vi "AA CH_LM App Main.vi"() -> ()   [LabVIEW 2012, in "CH_LM App.lvlib"]
doc: "This is the Main.vi of the LabMax PC Application."
uses:
  CH_LM App.lvlib
  CH_LM.lvlib
  CH_LM App FGV Functions.ctl
  _CH_LM/CH_LM FGV Functions.ctl
  CH_LM Globals Debug-Status.vi
panel:
  out "error":errorcluster
  in  "stop":bool
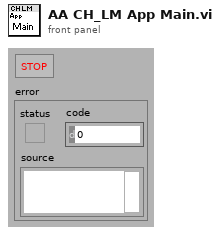
[diagram p1: front panel]
types:
  T1 = typedef "CH_LM.lvlib/CH_LM FGV Functions.ctl" = enum16{"create", "get", "set", "remove", "clear", "getBySerial"}
  T2 = typedef "CH_LM App.lvlib/CH_LM App FGV Functions.ctl" = enum16{"create", "get", "set", "remove", "clear", "getBySerial"}
  T3 = enum32{"Invalid", "Standard", "Closed", "Hidden", "Minimized", "Maximized"}
  T4 = enum32{"invalid app kind", "Development System", "Run Time System", "Student Edition", "Embedded LabVIEW", "Evaluation", "Custom"}
  T5 = typedef "LVRectTypeDef.ctl" = cluster{"Left":i16, "Top":i16, "Right":i16, "Bottom":i16}
  T6 = typedef "CH_LM.lvlib/CH_LM Communication Mode.ctl" = enum16{"None", "USB", "GPIB", "RS232"}
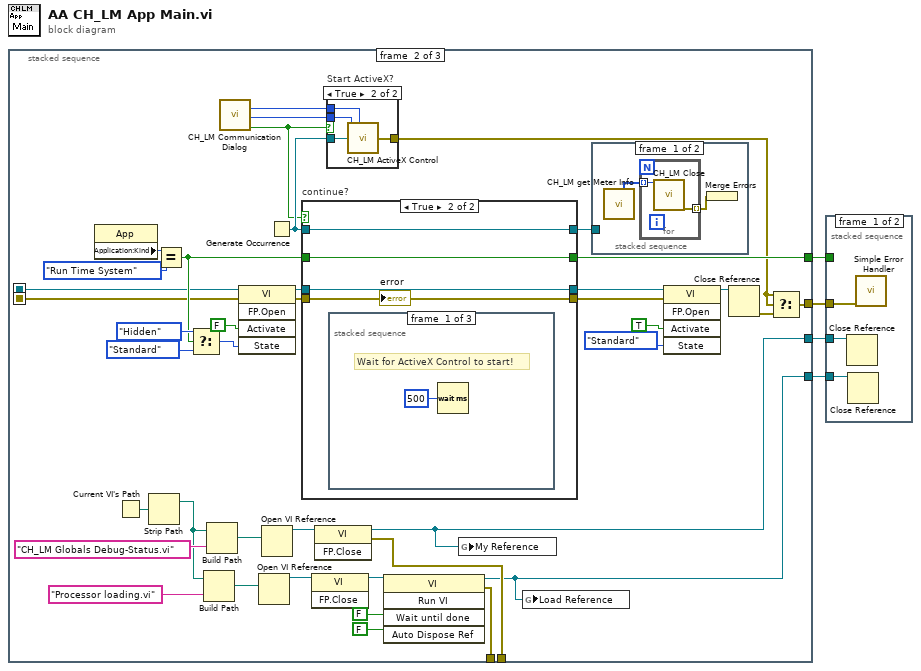
[diagram p0: block diagram]
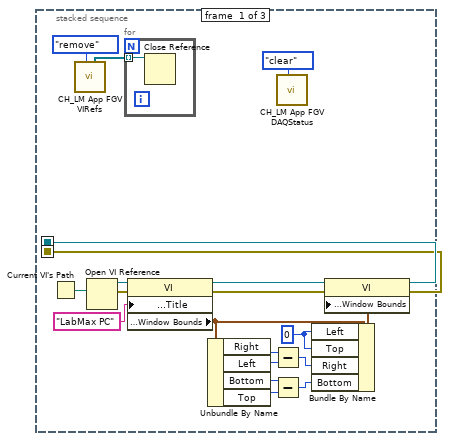
[diagram p2: hidden frame]
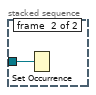
[diagram p3: hidden frame]
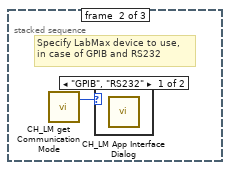
[diagram p6: hidden frame]
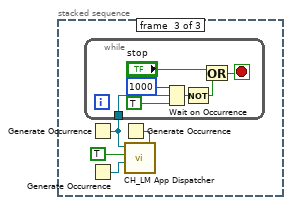
[diagram p8: hidden frame]
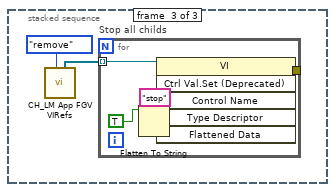
[diagram p9: hidden frame]
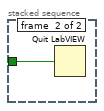
[diagram p10: hidden frame]
diagram:
  n1 = stacked-sequence {
    seq-local: [w15 _ _] -> [_ w43 _]
    seq-local: [w14 _ _] -> [_ w42 _]
    tunnel: [_ w62 _] -> w4
    tunnel: [_ w51 _] -> w3
    tunnel: [_ w36 _] -> w2
    tunnel: [_ w29 _] -> _
    tunnel: [_ w27 _] -> w1
    tunnel: [_ w28 _] -> _
    frame #0 {
      w6 = i16 0 ("left")
      n2 = Current VI's Path() -> (path=w18:path)
      n3 = call "CH_LM App FGV VIRefs.vi"("Function"=CH_LM_App_FGV_Functions."remove") -> ("VI Refs"=w23:refnum<vi>[])  [unwired: 3 in, 7 out]
      n4 = Open VI Reference(vi path=w18) -> (vi reference=w22:refnum<vi>, error out=w21:errorcluster)  [unwired: 1 in, 4 out]
      n5 = for {
        tunnel: w23 -> [w25] mode=indexing
        n6 = Close Reference(reference=w25) -> ()  [unwired: 1 in, 1 out]
      }
      n7 = property on="Property Node" class="VI"(reference=w22, error in=w21, "Front Panel Window:Title"="LabMax PC") -> (reference out=w17:refnum<vi>, error out=w16:errorcluster, "Front Panel Window:Window Bounds"=w19:T5)
      n8 = Unbundle By Name(w19) -> ("Right"=w7:i16, "Left"=w8:i16, "Bottom"=w10:i16, "Top"=w11:i16)
      n9 = Subtract(x=w7, y=w8) -> (x-y=w9:i16)
      n10 = Subtract(x=w10, y=w11) -> (x-y=w12:i16)
      n11 = call "CH_LM App FGV DAQStatus.vi"("Function"=CH_LM_FGV_Functions."clear") -> ()  [unwired: 3 in, 8 out]
      n12 = Bundle By Name(cluster=w19, "Left"=w6, "Top"=w6, "Right"=w9, "Bottom"=w12) -> (w5:T5)
      n13 = property on="Property Node" class="VI"(reference=w17, error in=w16, "Front Panel Window:Window Bounds"=w5) -> (reference out=w15:refnum<vi>, error out=w14:errorcluster)
    }
    frame #1 {
      n14 = property on="Property Node" class="App"() -> ("Application:Kind"=w65:T4)  [unwired: 2 in, 2 out]
      n15 = Current VI's Path() -> (path=w40:path)
      n16 = Strip Path(path=w40) -> (stripped path=w26:path)  [unwired: 1 out]
      n17 = Equal?(x=w65, y=T4."Run Time System" ("Application:Kind")) -> (x = y?=w44:bool)
      n18 = Select(t=T3."Hidden" ("State"), s=w44, f=T3."Standard" ("State")) -> (s? t:f=w46:T3)
      n19 = Build Path(base path=w26, name or relative path="Processor loading.vi") -> (appended path=w34:path)
      n20 = Build Path(base path=w26, name or relative path="CH_LM Globals Debug-Status.vi") -> (appended path=w38:path)
      n21 = call "CH_LM Communication Dialog.vi"() -> ("OK"=w48:bool, "Communication Mode"=w49:T6, "GPIB Board"=w50:i16)  [unwired: 5 out]
      n22 = invoke class="VI" method="FP.Open"(reference=w43, error in=w42, "Activate"=FALSE, "State"=w46) -> (reference out=w57:refnum<vi>, error out=w56:errorcluster)  [unwired: 1 in, 3 out]
      n23 = Open VI Reference(vi path=w34) -> (vi reference=w35:refnum<vi>)  [unwired: 5 in, 1 out]
      n24 = Open VI Reference(vi path=w38) -> (vi reference=w37:refnum<vi>)  [unwired: 5 in, 1 out]
      n25 = Generate Occurrence() -> (w63:refnum<k4>)
      n26 = case "continue?" shown="True" w48 {
        tunnel: w63 -> [w78 w82]
        tunnel: [w78 w82] -> w41
        tunnel: w44 -> [w75 w81]
        tunnel: [w75 w81] -> w62
        tunnel: w57 -> [w76 w80]
        tunnel: w56 -> [w77 w79]
        tunnel: [w76 w80] -> w55
        tunnel: [w77 w79] -> w54
        frame False {
        }
        frame True {
          n27 = stacked-sequence {
            frame #0 {
              # "Wait for ActiveX Control to start!"
              n28 = Wait (ms)(milliseconds to wait=u32 500) -> ()  [unwired: 1 out]
            }
            frame #1 {
              # "Specify LabMax device to use,\nin case of GPIB and RS232"
              n29 = call "CH_LM get Communication Mode.vi"() -> ("Communication Mode"=w84:T6)  [unwired: 1 in, 2 out]
              n30 = case shown="\"GPIB\", \"RS232\"" w84 {
                frame "GPIB", "RS232" {
                  n31 = call "CH_LM App Interface Dialog.vi"() -> ()  [unwired: 1 out]
                }
                frame Default {
                }
              }
            }
            frame #2 {
              n32 = Generate Occurrence() -> (w85:refnum<k4>)
              n33 = while {
                tunnel: w85 -> [w95]
                stop <- w89 stop-if-true
                n34 = Wait on Occurrence(1:TRUE ("ignore previous (T)"), 2:w95, 3:u32 1000 ("millisecond multiple")) -> (0:w94:bool)
                n35 = Not(x=w94) -> (.not. x?=w90:bool)
                n36 = Or(x="stop", y=w90) -> (x .or. y?=w89:bool)
              }
              n37 = Generate Occurrence() -> (w87:refnum<k4>)
              n38 = Generate Occurrence() -> (w86:refnum<k4>)
              n39 = call "CH_LM App Dispatcher.vi"("Menu occurrence"=w86, "Device disable occurrence"=w87, "MainGUI?"=TRUE, "Stop Main Occurrence"=w85) -> ()  [unwired: 1 in, 3 out]
            }
          }
          "error" <- w79
        }
      }
      n40 = invoke class="VI" method="FP.Close"(reference=w35) -> (reference out=w30:refnum<vi>)  [unwired: 2 in, 2 out]
      n41 = invoke class="VI" method="FP.Close"(reference=w37) -> (reference out=w36:refnum<vi>, error out=w29:errorcluster)  [unwired: 2 in, 1 out]
      n42 = case "Start ActiveX?" shown="True" w48 {
        tunnel: w63 -> [_ w74]
        tunnel: w50 -> [_ w73]
        tunnel: w49 -> [_ w72]
        tunnel: [_ w71] -> w52
        frame False {
        }
        frame True {
          n43 = call "CH_LM ActiveX Control.vi"("Communication Mode"=w72, "GPIB Board (0)"=w73, "MonitorStop Occurrence"=w74) -> ("error out"=w71:errorcluster)  [unwired: 1 in, 1 out]
        }
      }
      n44 = invoke class="VI" method="Run VI"(reference=w30, "Wait until done"=FALSE ("Wait Until Done"), "Auto Dispose Ref"=FALSE ("Auto Dispose Reference")) -> (reference out=w27:refnum<vi>, error out=w28:errorcluster)  [unwired: 2 in, 3 out]
      n45 = global write "CH_LM Globals Debug-Status.vi" "My Reference"(w36) -> ()
      n46 = global write "CH_LM Globals Debug-Status.vi" "Load Reference"(w27) -> ()
      n47 = stacked-sequence {
        tunnel: w41 -> [_ w70]
        frame #0 {
          n48 = call "CH_LM get Meter Info.vi"() -> ("All Meter Indices"=w67:i32[])  [unwired: 2 in, 9 out]
          n49 = for {
            tunnel: w67 -> [w69] mode=indexing
            tunnel: [w68] -> w66 mode=indexing
            n50 = call "CH_LM Close.vi"("Meter Index"=w69) -> ("error out"=w68:errorcluster)  [unwired: 1 in, 17 out]
          }
          n51 = Merge Errors(w66) -> ()  [unwired: 1 out]
        }
        frame #1 {
          n52 = Set Occurrence(w70) -> ()
        }
      }
      n53 = invoke class="VI" method="FP.Open"(reference=w55, error in=w54, "Activate"=TRUE, "State"=T3."Standard") -> (reference out=w58:refnum<vi>)  [unwired: 1 in, 4 out]
      n54 = Close Reference(reference=w58) -> (error out=w53:errorcluster)  [unwired: 1 in]
      n55 = Select(t=w52, s=w52, f=w53) -> (s? t:f=w51:errorcluster)
    }
    frame #2 {
      n56 = call "CH_LM App FGV VIRefs.vi"("Function"=CH_LM_App_FGV_Functions."remove") -> ("VI Refs"=w97:refnum<vi>[])  [unwired: 3 in, 7 out]
      n57 = for "Stop all childs" {
        tunnel: w97 -> [w103] mode=indexing
        tunnel: [w98] -> _
        n58 = Flatten To String(anything=TRUE) -> (data string=w100:string, type string=w101:i16[])  [unwired: 1 in, 3 out]
        n59 = invoke class="VI" method="Ctrl Val.Set (Deprecated)"(reference=w103, "Control Name"="stop", "Type Descriptor"=w101, "Flattened Data"=w100) -> (error out=w98:errorcluster)  [unwired: 2 in, 5 out]
      }
    }
  }
  n60 = stacked-sequence {
    tunnel: w4 -> [_ w107]
    tunnel: w3 -> [w106 _]
    tunnel: w2 -> [w105 _]
    tunnel: w1 -> [w104 _]
    frame #0 {
      n61 = Close Reference(reference=w105) -> ()  [unwired: 1 in, 1 out]
      n62 = Close Reference(reference=w104) -> ()  [unwired: 1 in, 1 out]
      n63 = call <vilib>:"Simple Error Handler.vi"("error in (no error)"=w106) -> ()  [unwired: 1 in, 8 out]
    }
    frame #1 {
      n64 = Quit LabVIEW(quit? (T)=w107) -> ()
    }
  }
